vi "Panel.vi"(11 "Game Config Panel in":refnum<class "Game Config Panel.lvclass">) -> ()   [LabVIEW 2020, in "SB App.lvlib" / "Game Config Panel.lvclass"]
uses:
  Game Config Panel.lvclass
  C:/Program Files (x86)/National Instruments/LabVIEW 2020/vi.lib/IlluminatedG/IG OOPanel/OOPanel/Panel/Panel.lvclass
  <vilib>/IlluminatedG/IG OOPanel/OOPanel/Panel/Basic UI State.ctl
  Game Config Panel.lvclass/Game Config Panel.ctl
  <vilib>/IlluminatedG/IG OOPanel/OOPanel/ArrayManager/ArrayManager.lvclass
  Game Start Data.ctl
  SquareBattle/Team Start Info.ctl
  SquareBattle/Team/Team.lvclass
  SquareBattle/Position.ctl
  Team Config Panel/Team Config Panel.lvclass
  C:/Program Files (x86)/National Instruments/LabVIEW 2020/vi.lib/IlluminatedG/IG OOPanel/OOPanel/ArrayPanel/ArrayPanel.lvclass
  <vilib>/IlluminatedG/IG OOPanel/OOPanel/Panel/Panel.lvclass
  <vilib>/IlluminatedG/IG OOPanel/OOPanel/OOPanel.lvlib
  SquareBattle/SquareBattle.lvlib
  SB App.lvlib
panel:
  in  "Random Starts":bool
  in  "Load":bool
  in  "Save":bool
  in  "Replication Rounds":u32=50
  in  "Board Size":i32=150
  in  "Add Team":bool
  in  "Start":bool
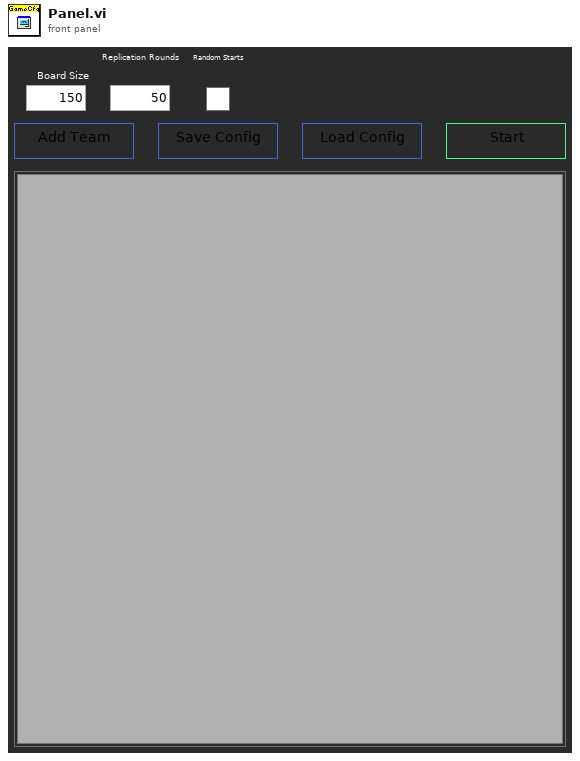
[diagram p1: front panel]
types:
  T1 = typedef "OOPanel.lvlib/Panel.lvclass/Basic UI State.ctl" = enum16{"Init", "Run", "Close"}
  T2 = enum8{"Enabled", "Disabled", "Disabled and Grayed Out"}
  T3 = typedef "SB App.lvlib/Game Start Data.ctl" = cluster{"Team Starts":T4[], "Board Size":i32, "Replication Rounds":u32}
  T4 = typedef "SquareBattle.lvlib/Team Start Info.ctl" = cluster{"Team":refnum<class "Team.lvclass">, "Position":T5}
  T5 = typedef "SquareBattle.lvlib/Position.ctl" = cluster{"Row":i32, "Col":i32}
  T6 = typedef "SB App.lvlib/Game Config Panel.lvclass/Incoming Events.ctl" = cluster{"Reset Config":refnum<user-event>, "Add Team":refnum<user-event>, "Start Position":refnum<user-event>}
  T7 = typedef "OOPanel.lvlib/Panel.lvclass/Panel Events.ctl" = cluster{"Visbility":refnum<user-event>, "Close":refnum<user-event>}
  T8 = typedef "SquareBattle.lvlib/Team ID.ctl" = u32
  T9 = map{T8, refnum<class "Team Config Panel.lvclass">}
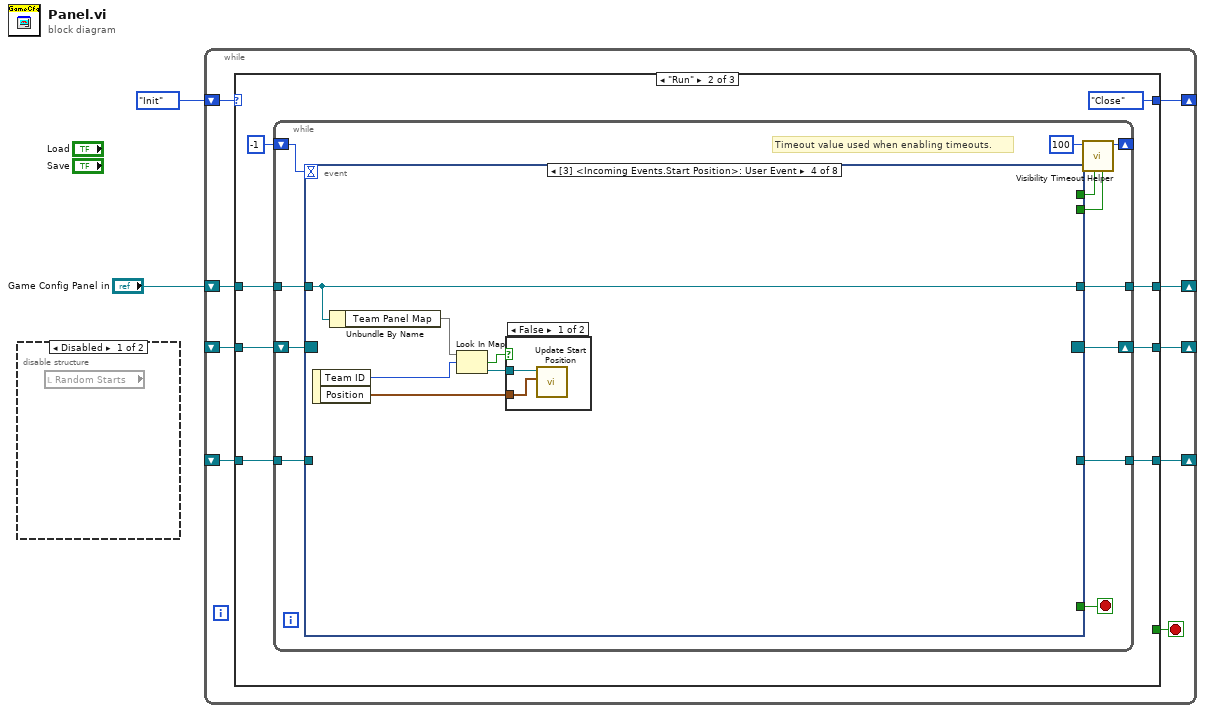
[diagram p0: block diagram]
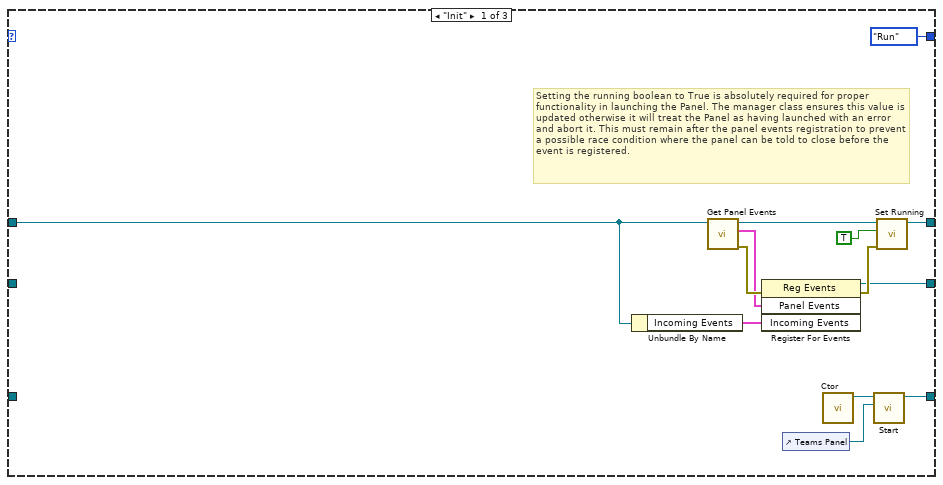
[diagram p3: hidden frame]
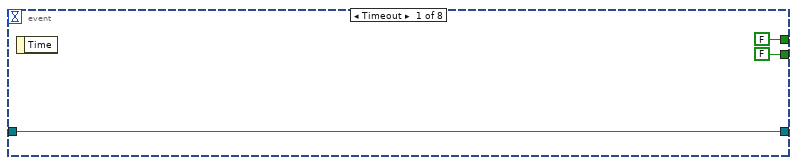
[diagram p4: hidden frame]
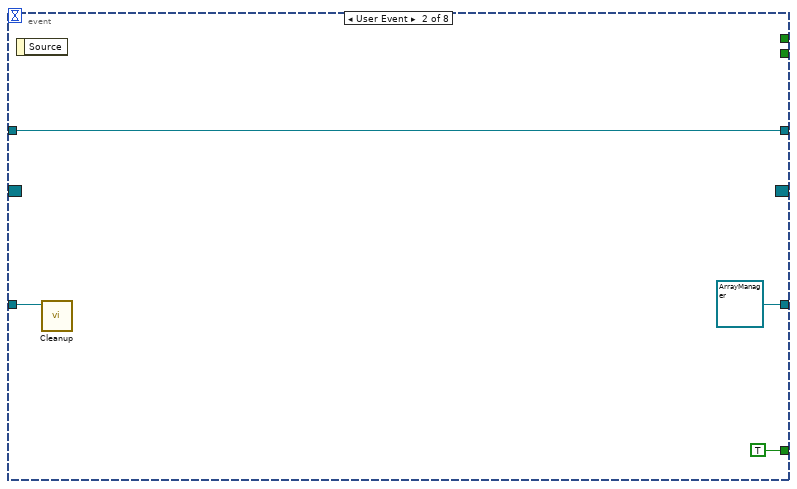
[diagram p5: hidden frame]
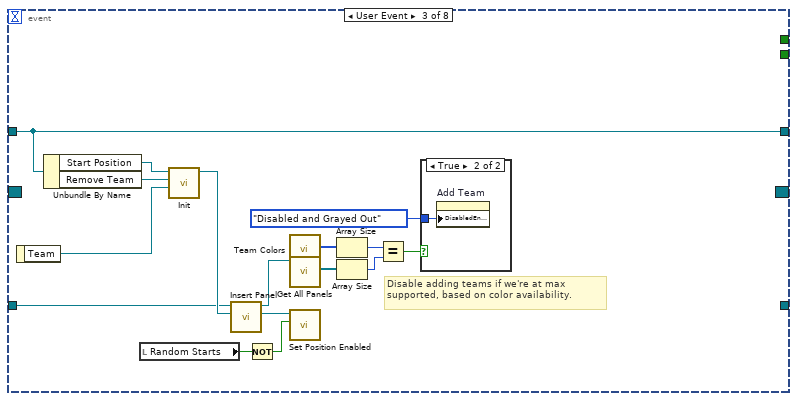
[diagram p6: hidden frame]
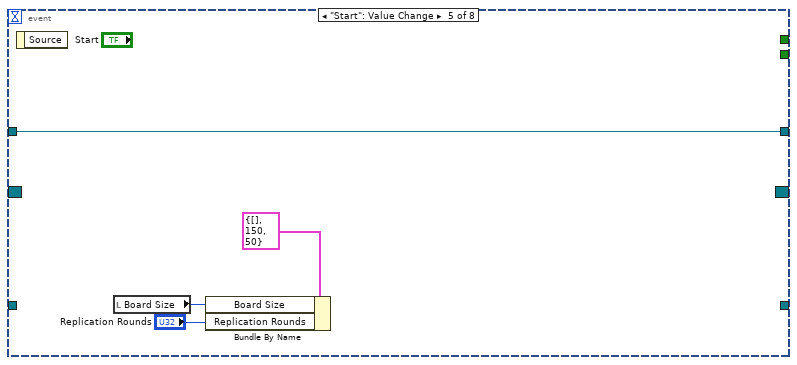
[diagram p9: hidden frame]
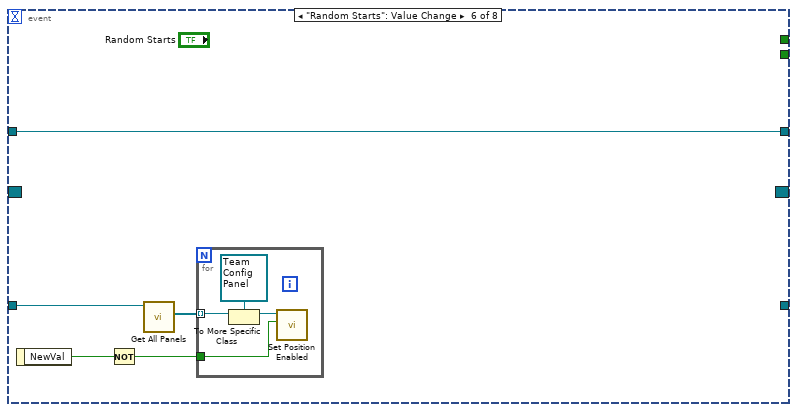
[diagram p10: hidden frame]
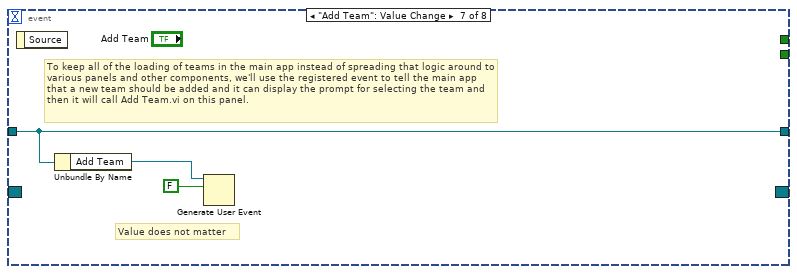
[diagram p11: hidden frame]
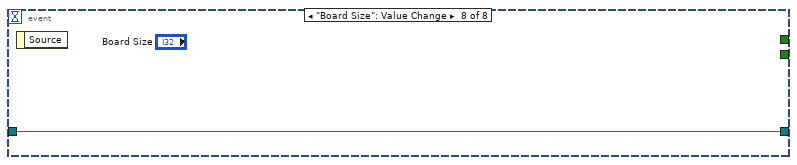
[diagram p12: hidden frame]
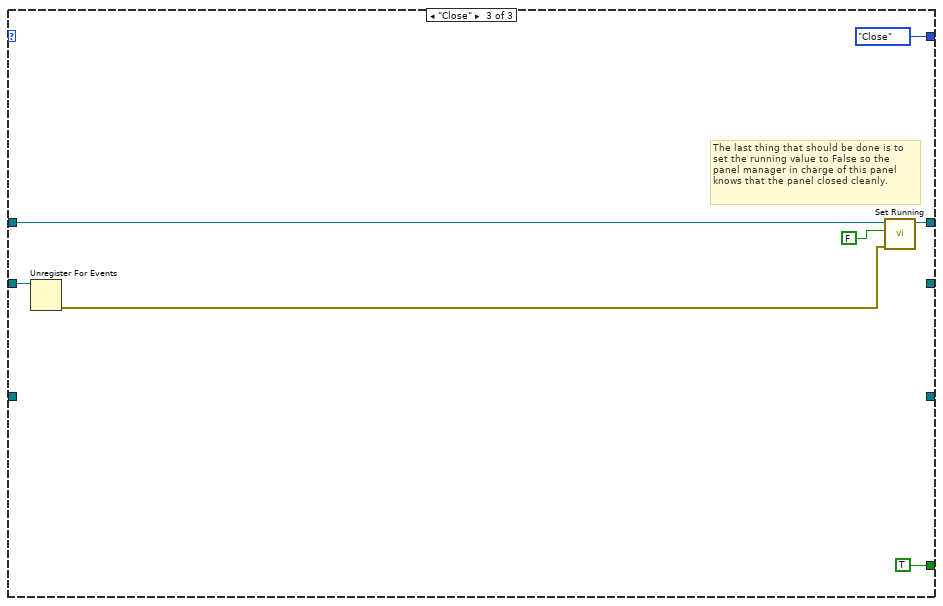
[diagram p13: hidden frame]
diagram:
  n1 = disable-structure shown="Disabled" {
    frame Disabled {
      n2 = local read "Random Starts"() -> ()  [unwired: 1 out]
    }
    frame Enabled {
    }
  }
  n3 = while {
    shift-right: [w10] -> _
    shift-left: _ -> [w11]
    shift-right: [w8] -> _
    shift-left: Basic_UI_State."Init" ("Basic UI State") -> [w9]
    shift-right: [w6] -> _
    shift-left: "Game Config Panel in" -> [w5]
    shift-right: [w4] -> _
    shift-left: _ -> [w3]
    stop <- w7 stop-if-true
    n4 = case shown="\"Run\"" w9 {
      tunnel: w11 -> [_ w32 w96]
      tunnel: [w18 w30 _] -> w10
      tunnel: [Basic_UI_State."Run" ("Basic UI State") Basic_UI_State."Close" ("Basic UI State") Basic_UI_State."Close" ("Basic UI State")] -> w8
      tunnel: [_ _ TRUE] -> w7
      tunnel: [w17 w27 w94] -> w6
      tunnel: w5 -> [w15 w28 w95]
      tunnel: [w12 w25 _] -> w4
      tunnel: w3 -> [_ w26 _]
      frame "Init" {
        # "Setting the running boolean to True is absolutely required for proper functionality in launching the Panel. The manager class ensures this value is updated otherwise it will treat the Panel as having launched with an error and abort it. This must remain after the panel events registration to prevent a possible race condition where the panel can be told to close before the event is registered."
        n5 = Unbundle By Name(w15) -> ("Incoming Events"=w16:T6)
        n6 = call <vilib>:"Get Panel Events.vi"("Panel in"=w15) -> ("error out"=w24:errorcluster, "Panel Events"=w20:T7, "Panel out"=w21:refnum<class "Game Config Panel.lvclass">)  [unwired: 8 in]
        n7 = register-events(error in=w24, w20, w16) -> (reference out=w18:refnum<event-registration>, error out=w22:errorcluster)  [unwired: 1 in]
        n8 = control-ref of="Teams Panel"() -> (w14:refnum<vi>)
        n9 = call <vilib>:"Ctor.vi"() -> ("PanelArray"=w13:refnum<class "ArrayManager.lvclass">)  [unwired: 10 in, 1 out]
        n10 = call <vilib>:"Start.vi"("Container"=w14, "ArrayManager in"=w13) -> ("ArrayManager out"=w12:refnum<class "ArrayManager.lvclass">)  [unwired: 8 in, 1 out]
        n11 = call <vilib>:"Set Running.vi"("error in (no error)"=w22, "Running"=TRUE, "Panel in"=w21) -> ("Panel out"=w17:refnum<class "Game Config Panel.lvclass">)  [unwired: 7 in, 1 out]
      }
      frame "Run" {
        n12 = while {
          shift-right: [w40] -> w30
          shift-left: w32 -> [w41]
          shift-right: [w43] -> _
          shift-left: -1 ("Timeout") -> [w42]
          tunnel: w28 -> [w36]
          tunnel: [w35] -> w27
          tunnel: w26 -> [w34]
          tunnel: [w33] -> w25
          stop <- w37 stop-if-true
          # "Timeout value used when enabling timeouts."
          n13 = event shown="[3] <Incoming Events.Start Position>: User Event" {
            selector: w41 -> [_ _ _ _ _ _ _ _]
            dyn-events: [_ _ _ _ _ _ _ _] -> w40
            timeout: w42 -> [_ _ _ _ _ _ _ _]
            tunnel: [FALSE _ _ _ _ _ _ _] -> w39
            tunnel: [FALSE _ _ _ _ _ _ _] -> w38
            tunnel: [_ TRUE _ _ _ _ _ _] -> w37
            tunnel: w36 -> [w45 w50 w67 w69 w77 w81 w92 w93]
            tunnel: [w45 w50 w67 w69 w77 w81 w92 w93] -> w35
            tunnel: w34 -> [_ w48 w59 _ _ w82 _ _]
            tunnel: [_ refnum<class "ArrayManager.lvclass"> refnum ("ArrayManager out") _ _ _ _ _ _] -> w33
            event Timeout {
              n14 = event-data() -> ()  [unwired: 1 in, 1 out]
            }
            event User Event {
              n15 = event-data() -> ()  [unwired: 1 in, 1 out]
              n16 = call <vilib>:"Cleanup.vi"("PanelArray in"=w48) -> ()  [unwired: 10 in, 1 out]
            }
            event User Event {
              # "Disable adding teams if we're at max supported, based on color availability."
              n17 = event-data() -> ("Team"=w65:refnum<class "Team.lvclass">)  [unwired: 1 in]
              n18 = Unbundle By Name(w67) -> ("Start Position"=w63:refnum<user-event>, "Remove Team"=w64:refnum<user-event>)
              n19 = local read "Random Starts"() -> (w61:bool)
              n20 = call "Init.vi"("Team"=w65, "Remove Team"=w64, "Start Position"=w63) -> ("Team Config Panel out"=w66:refnum<class "Team Config Panel.lvclass">)  [unwired: 7 in, 1 out]
              n21 = call <vilib>:"Insert Panel.vi"("Panel/Type"=w66, "PanelArray in"=w59) -> ("Panel"=w62:refnum<class "Team Config Panel.lvclass">, "PanelArray out"=w58:refnum<class "ArrayManager.lvclass">)  [unwired: 7 in, 1 out]
              n22 = Not(x=w61) -> (.not. x?=w60:bool)
              n23 = call "Team Colors.vi"() -> ("Team Colors"=w56:u32[])  [unwired: 11 in]
              n24 = call <vilib>:"Get All Panels.vi"("PanelArray in"=w58) -> ("Panels"=w57:refnum<class "ArrayPanel.lvclass">[])  [unwired: 8 in, 2 out]
              n25 = call "Set Position Enabled.vi"("Position Enabled"=w60, "Team Config Panel in"=w62) -> ()  [unwired: 8 in, 2 out]
              n26 = Array Size(array=w56) -> (size(s)=w55:i32)
              n27 = Array Size(array=w57) -> (size(s)=w54:i32)
              n28 = Equal?(x=w55, y=w54) -> (x = y?=w53:bool)
              n29 = case shown="True" w53 {
                tunnel: T2."Disabled and Grayed Out" ("Disabled") -> [_ w68]
                frame False {
                }
                frame True {
                  n30 = property on="Add Team" class="Bool"("DisabledEnum"=w68) -> ()  [unwired: 2 in, 2 out]
                }
              }
            }
            event User Event {
              n31 = event-data() -> ("Team ID"=w73:T8, "Position"=w72:T5)  [unwired: 1 in]
              n32 = Unbundle By Name(w69) -> ("Team Panel Map"=w74:T9)
              n33 = Look In Map(map=w74, key=w73) -> (key not found?=w71:bool, value=w70:refnum<class "Team Config Panel.lvclass">)  [unwired: 1 in]
              n34 = case shown="False" w71 {
                tunnel: w72 -> [w75 _]
                tunnel: w70 -> [w76 _]
                frame False {
                  n35 = call "Update Start Position.vi"("Position"=w75, "Team Config Panel in"=w76) -> ()  [unwired: 8 in, 2 out]
                }
                frame True {
                }
              }
            }
            event "Start": Value Change {
              n36 = event-data() -> ()  [unwired: 1 in, 1 out]
              n37 = local read "Board Size"() -> (w78:i32)
              n38 = Bundle By Name(cluster=T3 {"Team Starts"=[], "Board Size"=150, "Replication Rounds"=50} ("Game Start Data"), "Board Size"=w78, "Replication Rounds"="Replication Rounds") -> ()  [unwired: 1 out]
            }
            event "Random Starts": Value Change {
              n39 = event-data() -> ("NewVal"=w84:bool)  [unwired: 1 in]
              n40 = Not(x=w84) -> (.not. x?=w83:bool)
              n41 = call <vilib>:"Get All Panels.vi"("PanelArray in"=w82) -> ("Panels"=w85:refnum<class "ArrayPanel.lvclass">[])  [unwired: 8 in, 2 out]
              n42 = for {
                tunnel: w85 -> [w89] mode=indexing
                tunnel: w83 -> [w87]
                n43 = To More Specific Class(target class=refnum<class "Team Config Panel.lvclass"> refnum ("SB App.lvlib:Team Config Panel.lvclass"), reference=w89) -> (specific class reference=w86:refnum<class "Team Config Panel.lvclass">)  [unwired: 1 in, 1 out]
                n44 = call "Set Position Enabled.vi"("Position Enabled"=w87, "Team Config Panel in"=w86) -> ()  [unwired: 8 in, 2 out]
              }
            }
            event "Add Team": Value Change {
              # "Value does not matter"
              # "To keep all of the loading of teams in the main app instead of spreading that logic around to various panels and other components, we'll use the registered event to tell the main app that a new team should be added and it can display the prompt for selecting the team and then it will call Add Team.vi on this panel."
              n45 = event-data() -> ()  [unwired: 1 in, 1 out]
              n46 = Unbundle By Name(w92) -> ("Add Team"=w91:refnum<user-event>)
              n47 = Generate User Event(user event=w91, event data cluster=FALSE ("event data")) -> ()  [unwired: 2 in, 2 out]
            }
            event "Board Size": Value Change {
              n48 = event-data() -> ()  [unwired: 1 in, 1 out]
            }
          }
          n49 = call <vilib>:"Visibility Timeout Helper.vi"("Update?"=w38, "Use Timeout?"=w39, "Visible Timeout mS"=100) -> ("Timeout"=w43:i32)  [unwired: 8 in]
        }
      }
      frame "Close" {
        # "The last thing that should be done is to set the running value to False so the panel manager in charge of this panel knows that the panel closed cleanly."
        n50 = Unregister For Events(event registration refnum=w96) -> (error out=w98:errorcluster)  [unwired: 1 in]
        n51 = call <vilib>:"Set Running.vi"("error in (no error)"=w98, "Running"=FALSE, "Panel in"=w95) -> ("Panel out"=w94:refnum<class "Game Config Panel.lvclass">)  [unwired: 7 in, 1 out]
      }
    }
  }
